vi "TTA_MATLAB_TX_Perform1RFIC1TxOutputPowerTest.vi"(0 "Channel":string(combo), 1 "MXG VISA Resource In":refnum<visa-resource-name>, 2 "EXA VISA Resource":refnum<visa-resource-name>, 5 "Tx":string(combo), 11 "error in":errorcluster) -> (4 "Output Power\nResults":T1, 12 "MXG VISA Resource Out":refnum<visa-resource-name>, 13 "EXA VISA Resource Out":refnum<visa-resource-name>, 15 "error out":errorcluster)   [LabVIEW 2016]
uses:
  TTA_Globals/TTA_Global_Complete_Settings.vi
panel:
  out "End Temp":dbl
  out "Start Temp":dbl
  out "In Range?":bool[](array[boolean])
  out "Amp Max\nSpec (dBm)":dbl
  out "Amp Min\nSpec (dBm)":dbl
  out "Frequency":dbl[](array[numeric])
  out "Amplitude":dbl[](array[numeric])
  out "IF Index":i32
  in  "PALLinearization Values":T2
  out "Tx#":i32
  out "CH#":i32
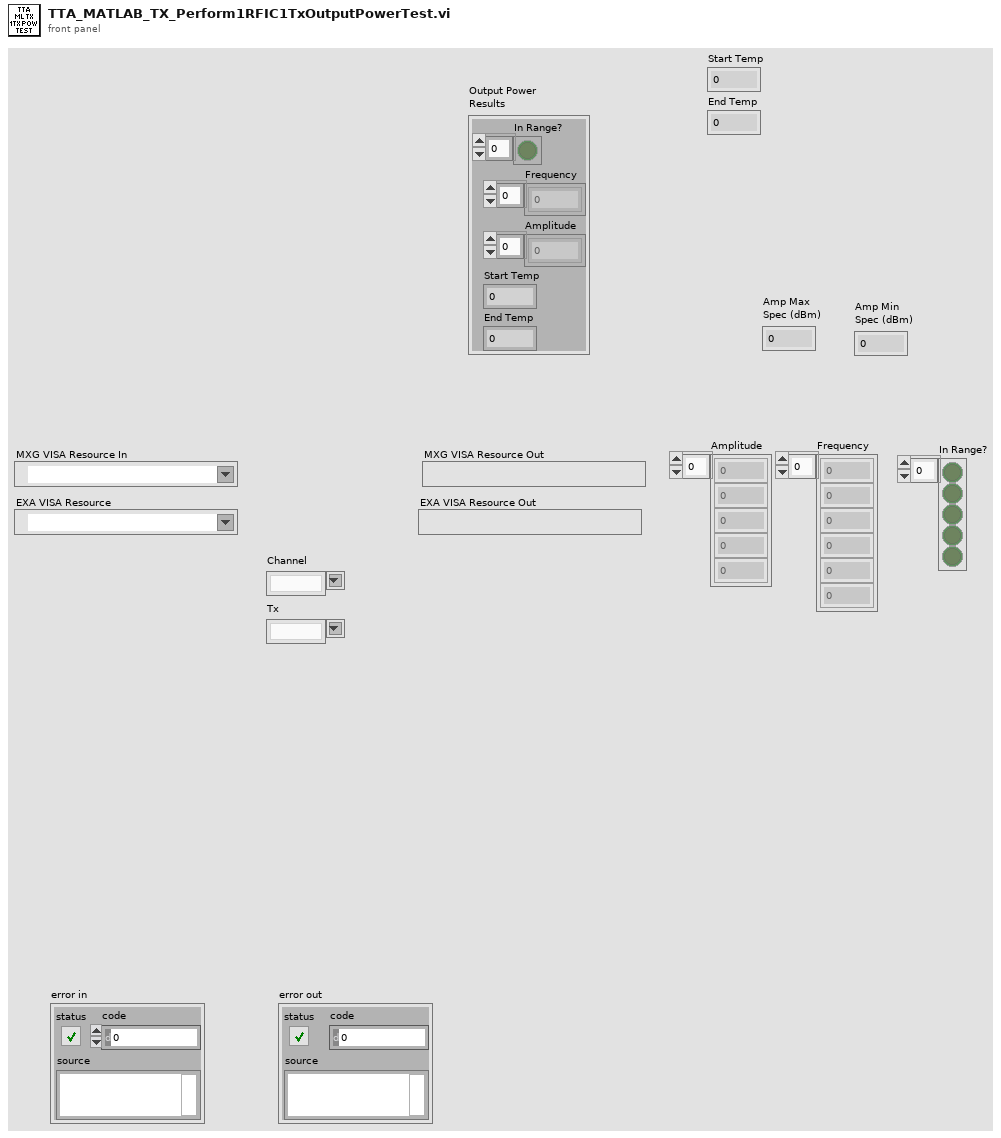
[diagram p1: front panel]
types:
  T1 = cluster{"In Range?":bool[], "Frequency":dbl[], "Amplitude":dbl[], "Start Temp":dbl, "End Temp":dbl}
  T2 = cluster{"Tx IF Offsets":dbl[], "ACPR Filename":string, "Sampling Rate":dbl, "TxIF_Freq":dbl, "Power (dBm)":dbl, "IF Frequency Sweep (MHz)":dbl[], "BDSFreq":dbl, "Amplitude Range\nMax(dBm)":dbl, "Amplitude Range\nMin(dBm)":dbl, "CAL Amplitude\nIncrement(dB)":dbl, "CAL Amplitude\nDecrement (dB)":dbl, "Amplitude Least\nCriteria (dBm)":dbl}
  T3 = typedef "TTA_Control_Complete_Settings_Cluster.ctl" = cluster{"Brief Cluster":cluster{"STM Firmware File":string, "STM Firmware Address":string, "Required SW Version":string, "Template Used":string}, "Instrument Setting Cluster":cluster{"BDSFreq":dbl, "BDS Amp":dbl, "TxRFCal_Freq":dbl, "TxRFCal_Amp":dbl, "RxRFCal_Freq":dbl, "RxRFCal_Freq":dbl, "TxIF_Freq":dbl, "TxIF_Amp":dbl, "Tx_Output_Power_Signal_Freq":dbl, "Tx_ACPR_Signal_Freq":dbl, "Rx_RF_Freq":dbl, "Rx_RF_Amp":dbl, "Rx_Output_Power_Signal_Freq":dbl, "Rx_Output_Power_Sense_Freq":dbl}, "PAL Calibration\nInputs Cluster":cluster{"Amplitude Range\nMax(dBm)":dbl, "Amplitude Range\nMin(dBm)":dbl, "Amplitude Least\nCriteria (dBm)":dbl, "Frequency 1":dbl, "Frequency 2":dbl, "Frequency 3":dbl, "CAL Amplitude\nDecrement (dB)":dbl, "CAL Amplitude\nIncrement(dB)":dbl, "DownloadFile":string}, "TxOffset Cal Cluster":cluster{"Tx1 Offset (dB)":dbl, "Tx2 Offset (dB)":dbl, "Tx3 Offset (dB)":dbl, "Tx4 Offset (dB)":dbl, "Total RF Tx Loss (dB)":dbl}, "RxOffset Cal Cluster":cluster{"Rx1 Offset (dB)":dbl, "Rx2 Offset (dB)":dbl, "Rx3 Offset (dB)":dbl, "Rx4 Offset (dB)":dbl, "Total RF Rx Loss (dB)":dbl}, "TX Output Power Settings Cluster":cluster{"Frequency Sweep (MHz)":dbl[], "Sig Gen \nPower (dBm)":dbl, "Span (kHz)":dbl, "RBW (Hz)":dbl, "Ref Level (dBm)":dbl, "Low Power \nLimit":dbl, "High Power \nLimit":dbl, "DigAtt Max":dbl, "DigAtt Min":dbl}, "Tx ACPR Settings Cluster":cluster{"ACPR Filename":string, "Sampling Rate":dbl, "Power (dBm)":dbl, "IF Frequency Sweep (MHz)":dbl[], "State Name":string, "Mechanical\nAttenuation":dbl, "RefLevel Offset":dbl, "Amplitude Range\nMax (dBm)":dbl, "Amplitude Range\nMin (dBm)":dbl, "Cal Amp \nIncrement (dB)":dbl, "Cal Amp\nDecrement (dB)":dbl}, "Power Cal Cluster":cluster{"Power List (dBm)":dbl[], "Frequency (MHz)":dbl[], "Cal Decrement (dB)":dbl, "Cal Increment (dB)":dbl}, "Rx Received Power Settings Cluster":cluster{"Frequency Sweep (MHz)":dbl[], "Power (dBm)":dbl, "Span (kHz)":dbl, "RBW (Hz)":dbl, "Ref Level":dbl, "Low Power \nLimit (dBm)":dbl, "High Power\nLimit (dBm)":dbl}, "Tx Output Power Criteria Cluster":cluster{"CH1-TX1 \nMin":dbl, "CH1-TX1\nMax":dbl, "CH1-TXx3\nMin ":dbl, "CH1-TXx3\nMax":dbl, "CH2-TX1\nMin":dbl, "CH2-TX1\nMax":dbl, "CH2-TXx3\nMin":dbl, "CH2-TXx3\nMax":dbl}, "Tx ACPR Criteria Cluster":cluster{"Min Inband":dbl, "Max Close Outband":dbl, "Max Far Outband":dbl}, "Rx Output Power Criteria Cluster":cluster{"CH1-RX1 \nMin":dbl, "CH1-RX1 \nMax":dbl, "CH1-RXx3 \nMin":dbl, "CH1-RXx3\nMax":dbl, "CH2-RX1\nMin":dbl, "CH2-RX1\nMax":dbl, "CH2-RXx3\nMin":dbl, "CH2-RXx3\nMax":dbl}}
  T4 = cluster{"BDSFreq":dbl, "BDS Amp":dbl, "TxRFCal_Freq":dbl, "TxRFCal_Amp":dbl, "RxRFCal_Freq":dbl, "RxRFCal_Freq":dbl, "TxIF_Freq":dbl, "TxIF_Amp":dbl, "Tx_Output_Power_Signal_Freq":dbl, "Tx_ACPR_Signal_Freq":dbl, "Rx_RF_Freq":dbl, "Rx_RF_Amp":dbl, "Rx_Output_Power_Signal_Freq":dbl, "Rx_Output_Power_Sense_Freq":dbl}
  T5 = cluster{"Tx1 Offset (dB)":dbl, "Tx2 Offset (dB)":dbl, "Tx3 Offset (dB)":dbl, "Tx4 Offset (dB)":dbl, "Total RF Tx Loss (dB)":dbl}
  T6 = cluster{"Frequency Sweep (MHz)":dbl[], "Sig Gen \nPower (dBm)":dbl, "Span (kHz)":dbl, "RBW (Hz)":dbl, "Ref Level (dBm)":dbl, "Low Power \nLimit":dbl, "High Power \nLimit":dbl, "DigAtt Max":dbl, "DigAtt Min":dbl}
  T7 = cluster{"CH1-TX1 \nMin":dbl, "CH1-TX1\nMax":dbl, "CH1-TXx3\nMin ":dbl, "CH1-TXx3\nMax":dbl, "CH2-TX1\nMin":dbl, "CH2-TX1\nMax":dbl, "CH2-TXx3\nMin":dbl, "CH2-TXx3\nMax":dbl}
  T8 = enum16{"TX1", "TX2", "TX3", "TX4", "TXx3", "TXx4", "RX1", "RX2", "RX3", "RX4", "RXx3", "RXx4", "RFCal"}
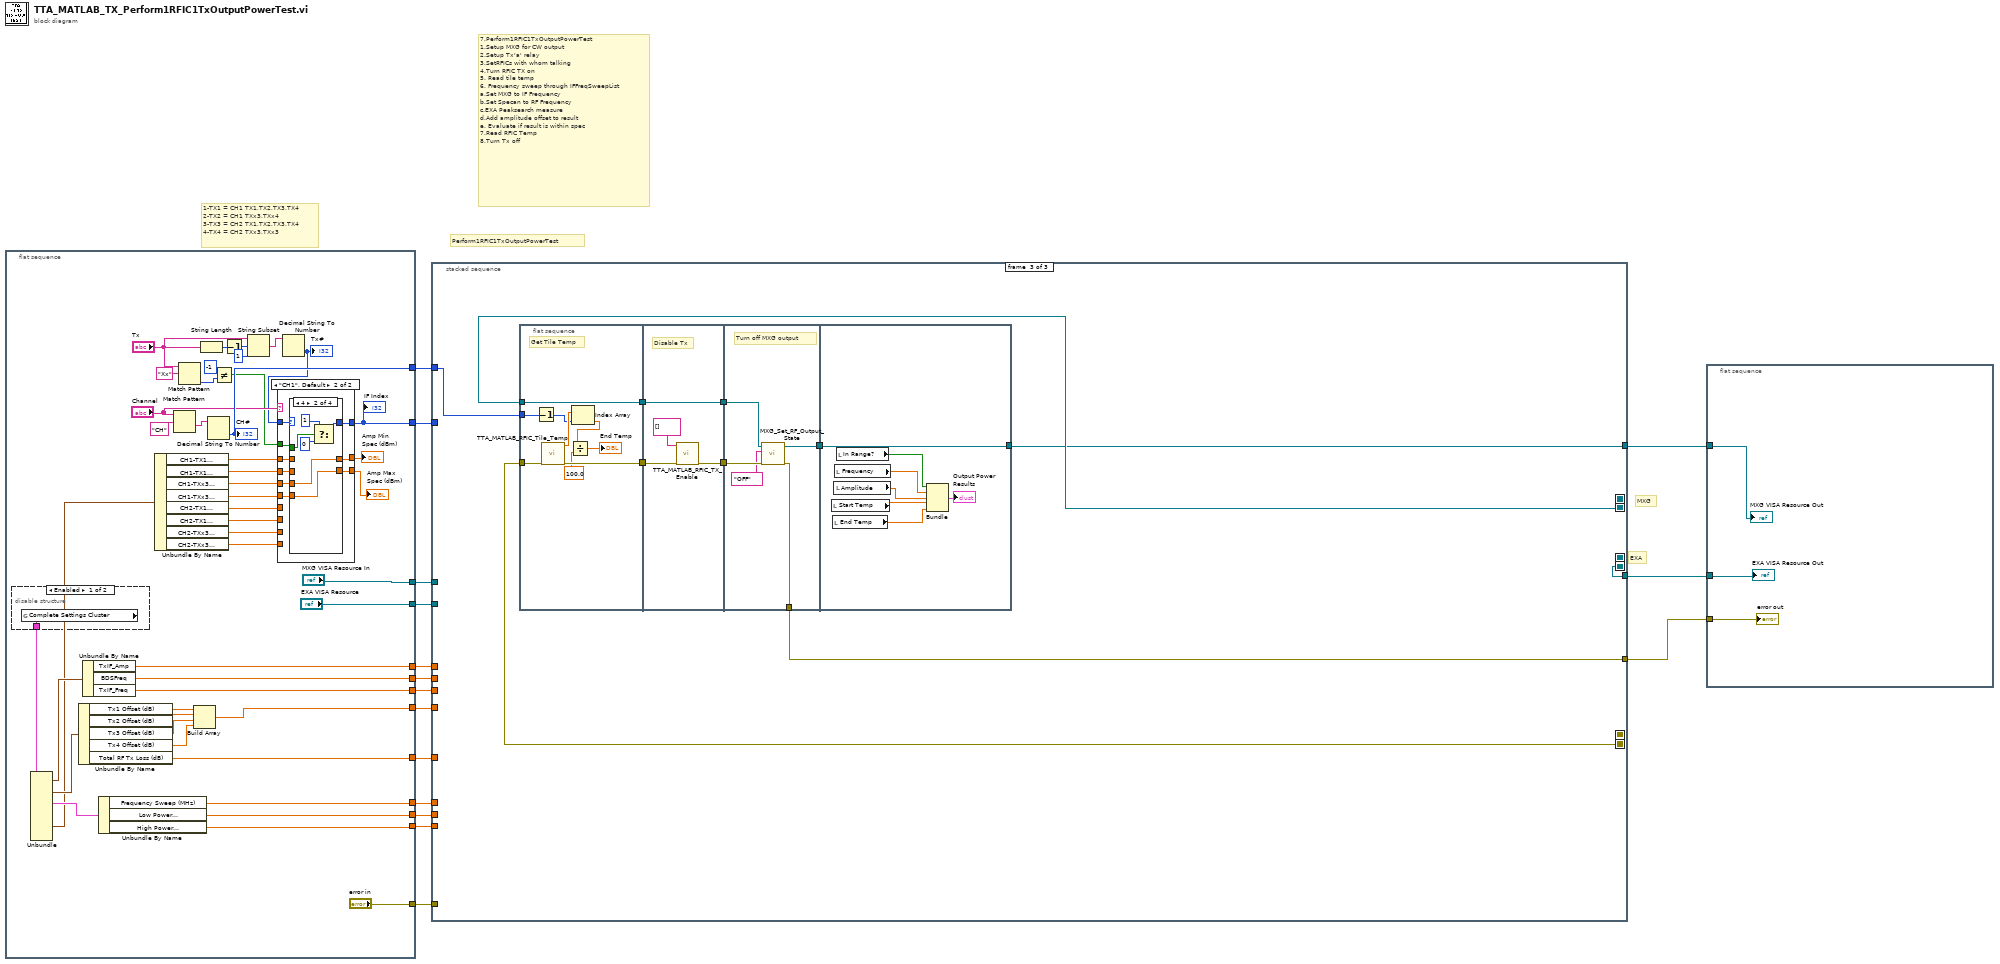
[diagram p0: block diagram]
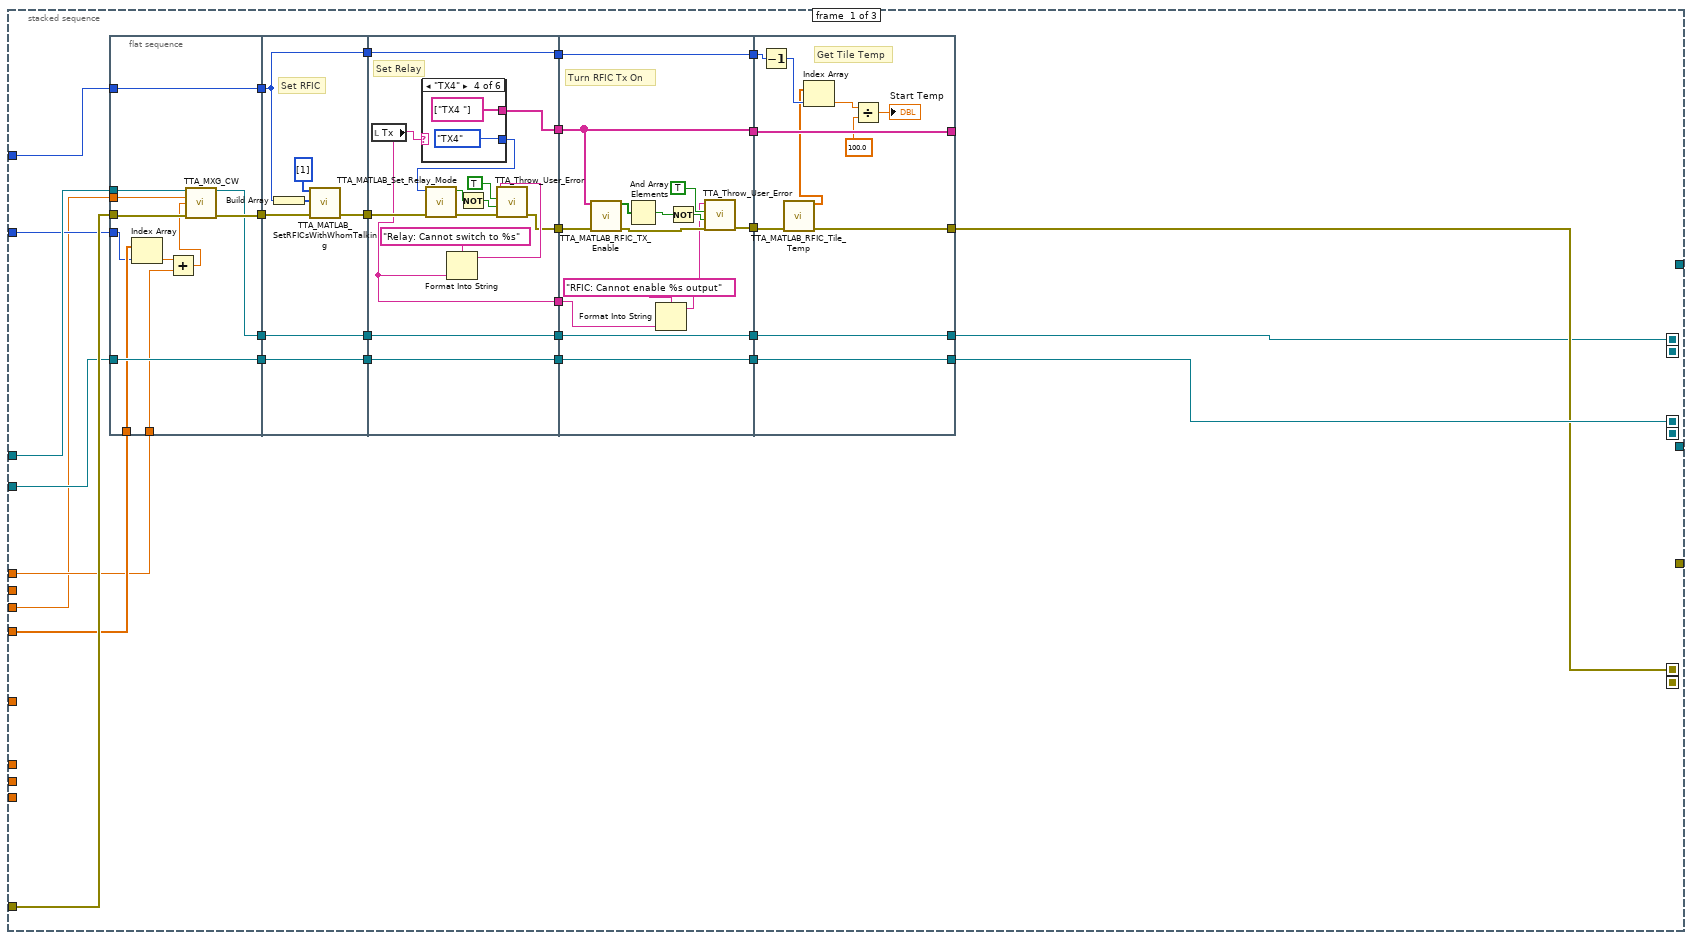
[diagram p2: hidden frame]
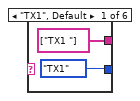
[diagram p3: hidden frame]
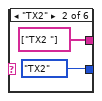
[diagram p4: hidden frame]
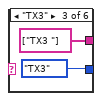
[diagram p5: hidden frame]
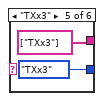
[diagram p6: hidden frame]
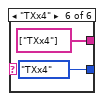
[diagram p7: hidden frame]
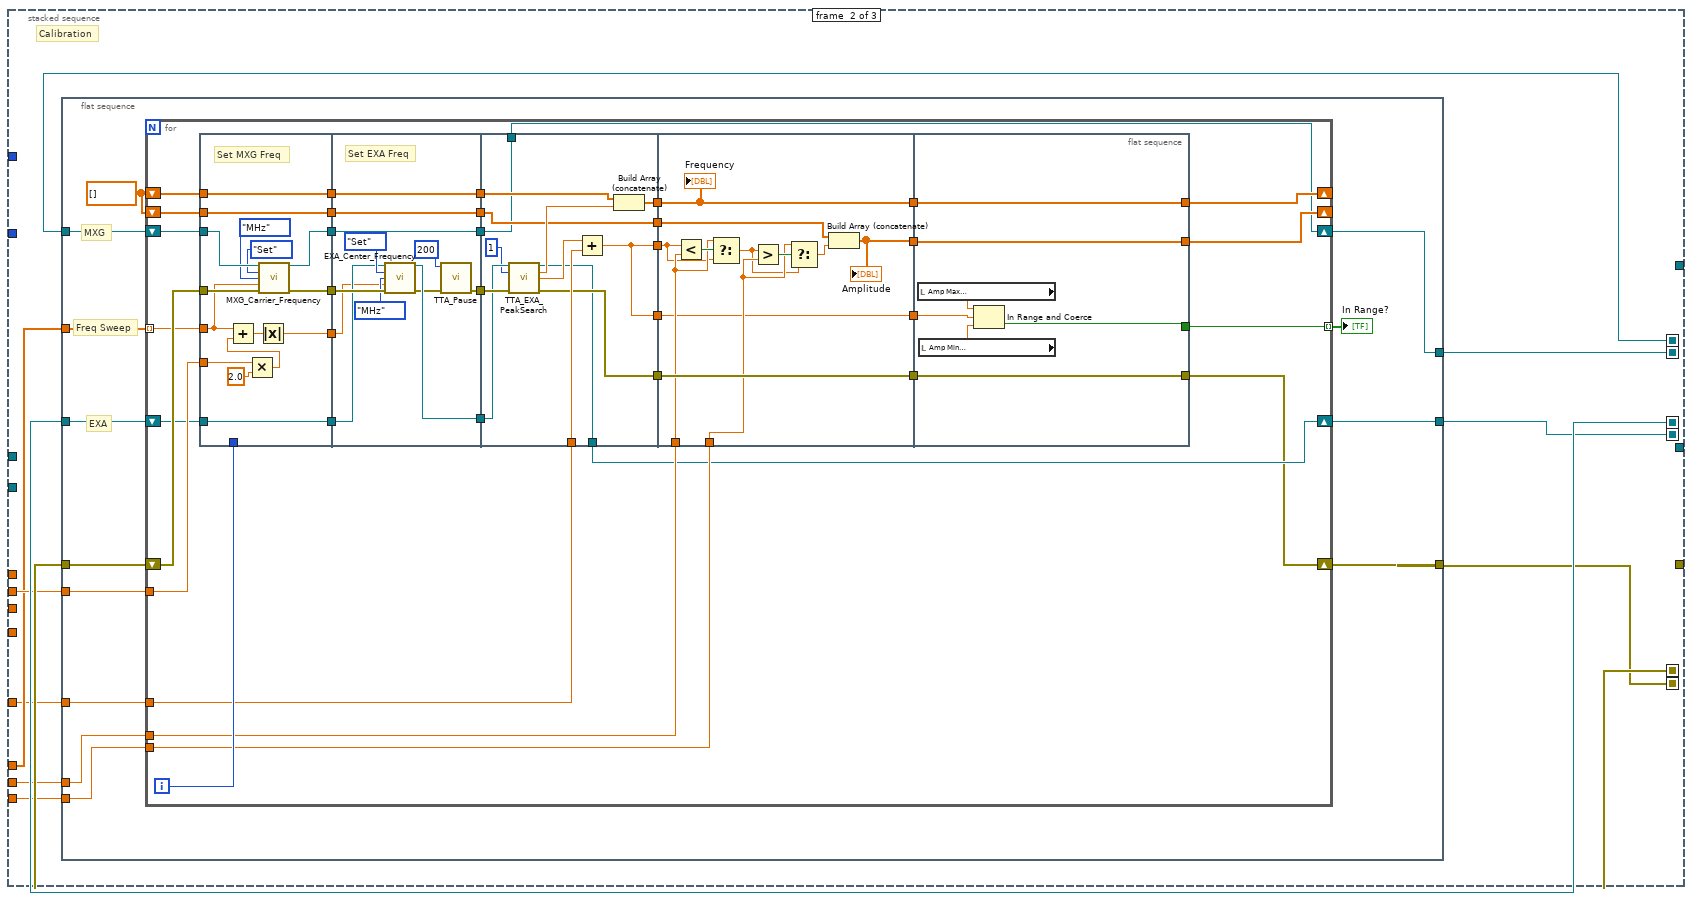
[diagram p8: hidden frame]
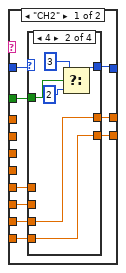
[diagram p9: hidden frame]
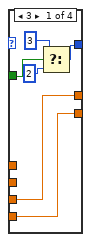
[diagram p10: hidden frame]
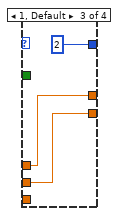
[diagram p11: hidden frame]
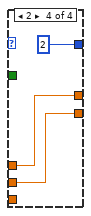
[diagram p12: hidden frame]
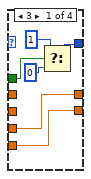
[diagram p13: hidden frame]
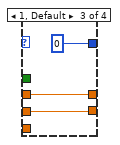
[diagram p14: hidden frame]
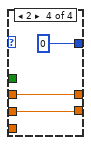
[diagram p15: hidden frame]
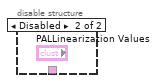
[diagram p16: hidden frame]
diagram:
  # "Perform1RFIC1TxOutputPowerTest"
  # "7.Perform1RFIC1TxOutputPowerTest\n1.Setup MXG for CW output\n2.Setup Tx'a' relay\n3.SetRFICs with whom talking\n4.Turn RFIC TX on\n5. Read tile temp\n6. Frequency sweep through IFFreqSweepList\na.Set MXG to IF Frequency\nb.Set Specan to RF Frequency\nc.EXA Peaksearch measure\nd.Add amplitude offset to result\ne. Evaluate if result is within spec\n7.Read RFIC Temp\n8.Turn Tx off"
  # "1-TX1 = CH1 TX1,TX2,TX3,TX4\n2-TX2 = CH1 TXx3,TXx4\n3-TX3 = CH2 TX1,TX2,TX3,TX4\n4-TX4 = CH2 TXx3,TXx3"
  # "EXA"
  # "MXG"
  n1 = flat-sequence {
    tunnel: ["error in"] -> w16
    tunnel: ["MXG VISA Resource In"] -> w14
    tunnel: ["EXA VISA Resource"] -> w13
    tunnel: [w56] -> w15
    tunnel: [w42] -> w10
    tunnel: [w43] -> w9
    tunnel: [w48] -> w8
    tunnel: [w34] -> w7
    tunnel: [w33] -> w6
    tunnel: [w31] -> w5
    tunnel: [w30] -> w4
    tunnel: [w29] -> w3
    tunnel: [w28] -> w2
    frame #0 {
      n2 = disable-structure shown="Enabled" {
        disable-tunnel: [w116 _] -> w51
        frame Enabled {
          n3 = global read "TTA_Global_Complete_Settings.vi" "Complete Settings Cluster"() -> (w116:T3)
        }
        frame Disabled {
        }
      }
      n4 = Unbundle(w51) -> ("Instrument Setting Cluster"=w50:T4, "TxOffset Cal Cluster"=w49:T5, "TX Output Power Settings Cluster"=w32:T6, "Tx Output Power Criteria Cluster"=w27:T7)  [unwired: 8 out]
      n5 = Unbundle By Name(w49) -> ("Tx1 Offset (dB)"=w47:dbl, "Tx2 Offset (dB)"=w46:dbl, "Tx3 Offset (dB)"=w45:dbl, "Tx4 Offset (dB)"=w44:dbl, "Total RF Tx Loss (dB)"=w30:dbl)
      n6 = Unbundle By Name(w50) -> ("TxIF_Amp"=w33:dbl, "BDSFreq"=w48:dbl, "TxIF_Freq"=w42:dbl)
      n7 = Unbundle By Name(w32) -> ("Frequency Sweep (MHz)"=w31:dbl[], "Low Power \nLimit"=w29:dbl, "High Power \nLimit"=w28:dbl)
      n8 = Unbundle By Name(w27) -> ("CH1-TX1 \nMin"=w26:dbl, "CH1-TX1\nMax"=w25:dbl, "CH1-TXx3\nMin"=w24:dbl, "CH1-TXx3\nMax"=w23:dbl, "CH2-TX1\nMin"=w22:dbl, "CH2-TX1\nMax"=w21:dbl, "CH2-TXx3\nMin"=w20:dbl, "CH2-TXx3\nMax"=w19:dbl)
      n9 = Match Pattern(string="Channel", regular expression="CH") -> (after substring=w57:string)  [unwired: 1 in, 3 out]
      n10 = Match Pattern(string="Tx", regular expression="Xx") -> (offset past match=w37:i32)  [unwired: 1 in, 3 out]
      n11 = Build Array(w47, w46, w45, w44) -> (w43:dbl[])
      n12 = String Length(string="Tx") -> (length=w55:i32)
      n13 = Decimal String To Number(string=w57) -> (number=w56:i32)  [unwired: 2 in, 1 out]
      "CH#" <- w56
      n14 = Not Equal?(x=-1, y=w37) -> (x != y?=w35:bool)
      n15 = Decrement(x=w55) -> (x-1=w54:i32)
      n16 = String Subset(string="Tx", offset (0)=w54, length (rest)=1 ("length (rest)")) -> (substring=w52:string)
      n17 = Decimal String To Number(string=w52) -> (number=w40:i32)  [unwired: 2 in, 1 out]
      "Tx#" <- w40
      n18 = case shown="\"CH1\", Default" "Channel" {
        tunnel: w40 -> [w69 w97]
        tunnel: [w70 w96] -> w34
        tunnel: w35 -> [w68 w95]
        tunnel: w26 -> [_ w94]
        tunnel: w25 -> [_ w93]
        tunnel: w24 -> [_ w92]
        tunnel: w23 -> [_ w91]
        tunnel: w22 -> [w67 _]
        tunnel: w21 -> [w66 _]
        tunnel: w20 -> [w65 _]
        tunnel: w19 -> [w64 _]
        tunnel: [w63 w90] -> w18
        tunnel: [w62 w89] -> w17
        frame "CH2" {
          n19 = case shown="4" w69 {
            tunnel: [w74 w80 2 2] -> w70
            tunnel: w68 -> [w73 w79 _ _]
            tunnel: w67 -> [_ _ w84 w87]
            tunnel: [w72 w78 w84 w87] -> w63
            tunnel: w66 -> [_ _ w83 w86]
            tunnel: [w71 w77 w83 w86] -> w62
            tunnel: w65 -> [w72 w78 _ _]
            tunnel: w64 -> [w71 w77 _ _]
            frame 3 {
              n20 = Select(t=3, s=w73, f=2) -> (s? t:f=w74:i32)
            }
            frame 4 {
              n21 = Select(t=3, s=w79, f=2) -> (s? t:f=w80:i32)
            }
            frame 1, Default {
            }
            frame 2 {
            }
          }
        }
        frame "CH1", Default {
          n22 = case shown="4" w97 {
            tunnel: [w101 w107 0 0] -> w96
            tunnel: w95 -> [w100 w106 _ _]
            tunnel: [w99 w105 w111 w114] -> w90
            tunnel: w94 -> [_ _ w111 w114]
            tunnel: [w98 w104 w110 w113] -> w89
            tunnel: w93 -> [_ _ w110 w113]
            tunnel: w92 -> [w99 w105 _ _]
            tunnel: w91 -> [w98 w104 _ _]
            frame 3 {
              n23 = Select(t=1, s=w100, f=0) -> (s? t:f=w101:i32)
            }
            frame 4 {
              n24 = Select(t=1, s=w106, f=0) -> (s? t:f=w107:i32)
            }
            frame 1, Default {
            }
            frame 2 {
            }
          }
        }
      }
      "IF Index" <- w34
      "Amp Min\nSpec (dBm)" <- w18
      "Amp Max\nSpec (dBm)" <- w17
    }
  }
  n25 = stacked-sequence {
    seq-local: [w121 _ _] -> [_ w227 _]
    seq-local: [w120 _ _] -> [_ w224 _]
    seq-local: [w134 _ _] -> [_ w226 _]
    seq-local: [_ w219 _] -> [_ _ w347]
    seq-local: [_ w217 _] -> [_ _ w344]
    seq-local: [_ w218 _] -> [_ _ w340]
    tunnel: w16 -> [w146 _ _]
    tunnel: w15 -> [w145 _ w337]
    tunnel: w14 -> [w143 _ _]
    tunnel: w13 -> [w142 _ _]
    tunnel: [_ _ w340] -> w12
    tunnel: [_ _ w339] -> w11
    tunnel: w10 -> [w126 _ _]
    tunnel: w9 -> [w128 _ _]
    tunnel: w8 -> [_ w225 _]
    tunnel: w7 -> [w129 _ _]
    tunnel: w6 -> [w127 _ _]
    tunnel: w5 -> [_ w223 _]
    tunnel: w4 -> [_ w222 _]
    tunnel: w3 -> [_ w221 _]
    tunnel: w2 -> [_ w220 _]
    tunnel: [_ _ w341] -> w1
    frame #0 {
      n26 = flat-sequence {
        tunnel: w142 -> [w157]
        tunnel: w143 -> [w154]
        tunnel: w145 -> [w158]
        tunnel: w146 -> [w156]
        tunnel: [w155] -> w133
        tunnel: [w158] -> w132
        tunnel: [w147] -> w131
        tunnel: [w157] -> w130
        tunnel: w129 -> [w152]
        tunnel: w128 -> [w153]
        tunnel: w127 -> [w151]
        tunnel: w126 -> [w148]
        tunnel: [w162] -> w144
        tunnel: [w161] -> w141
        tunnel: [w160] -> w140
        tunnel: w133 -> [w165]
        tunnel: w132 -> [w159]
        tunnel: w131 -> [w161]
        tunnel: w130 -> [w160]
        tunnel: [w159] -> w119
        tunnel: w144 -> [w179]
        tunnel: w141 -> [w171]
        tunnel: w140 -> [w169]
        tunnel: [w171] -> w139
        tunnel: [w167] -> w138
        tunnel: [w170] -> w137
        tunnel: [w169] -> w136
        tunnel: [w168] -> w135
        tunnel: w119 -> [w166]
        tunnel: [w166] -> w118
        tunnel: w139 -> [w194]
        tunnel: w138 -> [w198]
        tunnel: w137 -> [w197]
        tunnel: w136 -> [w196]
        tunnel: w135 -> [w195]
        tunnel: [w196] -> w125
        tunnel: [w198] -> w124
        tunnel: [w194] -> w123
        tunnel: [w193] -> w122
        tunnel: w118 -> [w192]
        tunnel: [w192] -> w117
        tunnel: [w214] -> w120
        tunnel: [w215] -> _
        tunnel: [w216] -> w134
        tunnel: w125 -> [w216]
        tunnel: w124 -> [w215]
        tunnel: w123 -> [w214]
        tunnel: w122 -> [w213]
        tunnel: [w212] -> w121
        tunnel: w117 -> [w210]
        frame #0 {
          n27 = Index Array(array=w153, index=w152) -> (element=w150:dbl)
          n28 = Add(x=w150, y=w151) -> (x+y=w149:dbl)
          n29 = call "TTA_MXG_CW.vi"("VISA resource In"=w154, "Frequency (MHz)"=w148, "Output Power\nLevel (dBm)"=w149, "error in"=w156) -> ("VISA resource Out"=w147:refnum<visa-resource-name>, "error out"=w155:errorcluster)  [unwired: 10 in]
        }
        frame #1 {
          # "Set RFIC"
          n30 = Build Array(w159) -> (w163:i32[])
          n31 = call "TTA_MATLAB_SetRFICsWithWhomTalking.vi"("Panel Array"=i32[] [1], "RFIC Array"=w163, "error in"=w165) -> ("error out"=w162:errorcluster)  [unwired: 12 in]
        }
        frame #2 {
          # "Set Relay"
          n32 = local read "Tx"() -> (w168:string)
          n33 = case shown="\"TX4\"" w168 {
            tunnel: [T8."TX1" ("Mode") T8."TX2" ("Mode") T8."TX3" ("Mode") T8."TX4" ("Mode") T8."TXx3" ("Mode") T8."TXx4" ("Mode")] -> w178
            tunnel: [string[] ["TX1 "] ("Channels") string[] ["TX2 "] ("Channels") string[] ["TX3 "] ("Channels") string[] ["TX4 "] ("Channels") string[] ["TXx3"] ("Channels") string[] ["TXx4"] ("Channels")] -> w167
            frame "TX1", Default {
            }
            frame "TX2" {
            }
            frame "TX3" {
            }
            frame "TX4" {
            }
            frame "TXx3" {
            }
            frame "TXx4" {
            }
          }
          n34 = call "TTA_MATLAB_Set_Relay_Mode.vi"("error in"=w179, "Mode"=w178) -> ("error out"=w177:errorcluster, "Success"=w176:bool)  [unwired: 8 in]
          n35 = Format Into String(format string="Relay: Cannot switch to %s", w168) -> (resulting string=w172:string)  [unwired: 2 in, 1 out]
          n36 = Not(x=w176) -> (.not. x?=w175:bool)
          n37 = call "TTA_Throw_User_Error.vi"("error in"=w177, "Error?"=w175, "Stop Execution on Fail"=TRUE, "Error Message"=w172) -> ("error out"=w170:errorcluster)  [unwired: 7 in]
        }
        frame #3 {
          # "Turn RFIC Tx On"
          n38 = call "TTA_MATLAB_RFIC_TX_Enable.vi"("Channels"=w198, "error in"=w197) -> ("SuccessComm"=w205:bool[], "error out"=w201:errorcluster)  [unwired: 12 in]
          n39 = And Array Elements(Boolean array=w205) -> (logical AND=w202:bool)
          n40 = Format Into String(format string="RFIC: Cannot enable %s output", w195) -> (resulting string=w199:string)  [unwired: 2 in, 1 out]
          n41 = Not(x=w202) -> (.not. x?=w203:bool)
          n42 = call "TTA_Throw_User_Error.vi"("error in"=w201, "Error?"=w203, "Stop Execution on Fail"=TRUE, "Error Message"=w199) -> ("error out"=w193:errorcluster)  [unwired: 7 in]
        }
        frame #4 {
          # "Get Tile Temp"
          n43 = Decrement(x=w210) -> (x-1=w209:i32)
          n44 = call "TTA_MATLAB_RFIC_Tile_Temp.vi"("error in"=w213) -> ("Results"=w208:dbl[], "error out"=w212:errorcluster)  [unwired: 11 in, 2 out]
          n45 = Index Array(array=w208, index=w209) -> (element=w207:dbl)
          n46 = Divide(x=w207, y=100.0) -> (x/y=→"Start Temp":dbl)
        }
      }
    }
    frame #1 {
      # "Calibration"
      n47 = flat-sequence {
        tunnel: w227 -> [w240]
        tunnel: w226 -> [w239]
        tunnel: [w238] -> w218
        tunnel: [w237] -> w219
        tunnel: w225 -> [w236]
        tunnel: w223 -> [w235]
        tunnel: w224 -> [w234]
        tunnel: w222 -> [w233]
        tunnel: w221 -> [w231]
        tunnel: w220 -> [w230]
        tunnel: [w229] -> w217
        frame #0 {
          w232 = dbl[] []
          # "Freq Sweep"
          # "EXA"
          # "MXG"
          n48 = for {
            shift-right: [w247] -> w237
            shift-left: w240 -> [w274]
            shift-right: [w248] -> w238
            shift-left: w239 -> [w273]
            tunnel: w236 -> [w276]
            tunnel: w235 -> [w272] mode=indexing
            shift-right: [w249] -> w229
            shift-left: w234 -> [w275]
            tunnel: w233 -> [w264]
            shift-right: [w263] -> _
            shift-left: w232 -> [w258]
            shift-right: [w262] -> _
            shift-left: w232 -> [w261]
            tunnel: w231 -> [w253]
            tunnel: w230 -> [w252]
            tunnel: [w241] -> w228 mode=indexing
            i -> [w277]
            n49 = flat-sequence {
              tunnel: w272 -> [w284]
              tunnel: w277 -> [_]
              tunnel: w276 -> [w288]
              tunnel: w275 -> [w291]
              tunnel: w274 -> [w292]
              tunnel: w273 -> [w281]
              tunnel: [w283] -> w271
              tunnel: [w282] -> w270
              tunnel: [w281] -> w269
              tunnel: [w280] -> w268
              tunnel: w261 -> [w279]
              tunnel: [w279] -> w259
              tunnel: w258 -> [w278]
              tunnel: [w278] -> w256
              tunnel: w271 -> [w300]
              tunnel: w270 -> [w304]
              tunnel: w269 -> [w302]
              tunnel: w268 -> [w298]
              tunnel: [w299] -> w267
              tunnel: [w298] -> w266
              tunnel: [w295] -> w265
              tunnel: [w294] -> w260
              tunnel: w259 -> [w294]
              tunnel: [w293] -> w257
              tunnel: w256 -> [w293]
              tunnel: w267 -> [w316]
              tunnel: w266 -> [w307]
              tunnel: w265 -> [w317]
              tunnel: w264 -> [w314]
              tunnel: w260 -> [w310]
              tunnel: w257 -> [w309]
              tunnel: [w312] -> w255
              tunnel: [w305] -> w254
              tunnel: [w309] -> w251
              tunnel: [w308] -> w250
              tunnel: [w307] -> w249
              tunnel: [w306] -> w248
              tunnel: [w305] -> w242
              tunnel: w255 -> [w329]
              tunnel: w254 -> [w326]
              tunnel: w253 -> [w327]
              tunnel: w252 -> [w324]
              tunnel: w251 -> [w321]
              tunnel: w250 -> [w319]
              tunnel: [w329] -> w246
              tunnel: [w319] -> w245
              tunnel: [w320] -> w244
              tunnel: [w318] -> w243
              tunnel: w242 -> [w318]
              tunnel: [w334] -> w263
              tunnel: [w335] -> w262
              tunnel: [w336] -> w247
              tunnel: w246 -> [w336]
              tunnel: w245 -> [w335]
              tunnel: w244 -> [w334]
              tunnel: w243 -> [w331]
              tunnel: [w330] -> w241
              frame #0 {
                # "Set MXG Freq"
                n50 = Multiply(x=w288, y=2.0) -> (x*y=w286:dbl)
                n51 = Add(x=w284, y=w286) -> (x+y=w285:dbl)
                n52 = Absolute Value(x=w285) -> (abs(x)=w283:dbl)
                n53 = call "MXG_Carrier_Frequency.vi"("VISA resource name"=w291, "Mode"=enum16{"Set", "Get"}."Set", "Units"=enum16{"Hz", "kHz", "MHz", "GHz"}."MHz", "Frequency"=w284, "error in"=w292) -> ("VISA resource name"=w280:refnum<visa-resource-name>, "error out"=w282:errorcluster)  [unwired: 8 in, 1 out]
              }
              frame #1 {
                # "Set EXA Freq"
                n54 = call "EXA_Center_Frequency.vi"("VISA resource name"=w302, "Mode"=enum16{"Set", "Get"}."Set", "Units"=enum16{"Hz", "kHz", "MHz", "GHz"}."MHz", "Frequency"=w300, "error in"=w304) -> ("VISA resource name"=w299:refnum<visa-resource-name>, "error out"=w297:errorcluster)  [unwired: 8 in, 1 out]
                n55 = call "TTA_Pause.vi"("error in"=w297, "Pause (ms)"=u32 200) -> ("error out"=w295:errorcluster)  [unwired: 9 in]
              }
              frame #2 {
                n56 = call "TTA_EXA_PeakSearch.vi"("VISA resource In"=w316, "Marker\nNumber"=1 ("Marker\nNumber"), "error in"=w317) -> ("VISA resource Out"=w306:refnum<visa-resource-name>, "Frequency (Hz)"=w311:dbl, "Amplitude (dBm)"=w313:dbl, "error out"=w312:errorcluster)  [unwired: 9 in]
                n57 = Add(x=w313, y=w314) -> (x+y=w305:dbl)
                n58 = Build Array (concatenate)(w310, w311) -> (w308:dbl[])
              }
              frame #3 {
                n59 = Less?(x=w326, y=w327) -> (x < y?=w328:bool)
                n60 = Select(t=w327, s=w328, f=w326) -> (s? t:f=w323:dbl)
                n61 = Greater?(x=w323, y=w324) -> (0:w325:bool)
                n62 = Select(t=w324, s=w325, f=w323) -> (s? t:f=w322:dbl)
                n63 = Build Array (concatenate)(w321, w322) -> (w320:dbl[])
                "Amplitude" <- w320
                "Frequency" <- w319
              }
              frame #4 {
                n64 = local read "Amp Max\nSpec (dBm)"() -> (w333:dbl)
                n65 = local read "Amp Min\nSpec (dBm)"() -> (w332:dbl)
                n66 = In Range and Coerce(upper limit=w333, x=w331, lower limit=w332) -> (In Range?=w330:bool)  [unwired: 1 out]
              }
            }
          }
          "In Range?" <- w228
        }
      }
    }
    frame #2 {
      n67 = flat-sequence {
        tunnel: w347 -> [w354]
        tunnel: [w356] -> w346
        tunnel: w344 -> [w353]
        tunnel: [w353] -> w342
        tunnel: w337 -> [w352]
        tunnel: w346 -> [w359]
        tunnel: [w358] -> w345
        tunnel: [w357] -> w343
        tunnel: w342 -> [w357]
        tunnel: w345 -> [w365]
        tunnel: w343 -> [w364]
        tunnel: [w361] -> w339
        tunnel: [w362] -> w338
        tunnel: [w372] -> w341
        tunnel: w338 -> [w372]
        frame #0 {
          # "Get Tile Temp"
          n68 = Decrement(x=w352) -> (x-1=w350:i32)
          n69 = call "TTA_MATLAB_RFIC_Tile_Temp.vi"("error in"=w354) -> ("Results"=w351:dbl[], "error out"=w356:errorcluster)  [unwired: 11 in, 2 out]
          n70 = Index Array(array=w351, index=w350) -> (element=w349:dbl)
          n71 = Divide(x=w349, y=100.0) -> (x/y=→"End Temp":dbl)
        }
        frame #1 {
          # "Disable Tx"
          n72 = call "TTA_MATLAB_RFIC_TX_Enable.vi"("Channels"=string[] [], "error in"=w359) -> ("error out"=w358:errorcluster)  [unwired: 12 in, 1 out]
        }
        frame #2 {
          # "Turn off MXG output"
          n73 = call "MXG_Set_RF_Output_State.vi"("error in"=w365, "RF Output State"="OFF", "VISA resource name"=w364) -> ("error out"=w361:errorcluster, "VISA resource name"=w362:refnum<visa-resource-name>)  [unwired: 7 in]
        }
        frame #3 {
          n74 = local read "Start Temp"() -> (w368:dbl)
          n75 = local read "End Temp"() -> (w367:dbl)
          n76 = local read "Amplitude"() -> (w369:dbl[])
          n77 = local read "Frequency"() -> (w370:dbl[])
          n78 = local read "In Range?"() -> (w371:bool[])
          n79 = Bundle("In Range?"=w371, "Frequency"=w370, "Amplitude"=w369, "Start Temp"=w368, "End Temp"=w367) -> (→"Output Power\nResults":T1)  [unwired: 1 in]
        }
      }
    }
  }
  n80 = flat-sequence {
    tunnel: w12 -> [w375]
    tunnel: w11 -> [w374]
    tunnel: w1 -> [w373]
    frame #0 {
      "error out" <- w374
      "MXG VISA Resource Out" <- w373
      "EXA VISA Resource Out" <- w375
    }
  }
